vi "CompensateTRY.vi"(0 "Right Wheel Setpoint":dbl, 1 "LeftDriveRefNum":string="My Encoder RefNum", 2 "Try":bool, 3 "Left Wheel Setpoint":dbl, 4 "RightDriveRefNum":string="My Encoder RefNum") -> (5 "Right Wheel Setpoint Out":dbl, 7 "Left Wheel Setpoint Out":dbl)   [LabVIEW 2014]
uses:
  <vilib>/addons/control/pid/pid.llb/PID (DBL).vi
  <vilib>/addons/control/pid/NI_PID_pid.lvlib
panel:
  out "compensate 2":dbl(graph)
  out "compensate 1":dbl(graph)
  out "Dist 2":dbl(graph)
  out "Dist 1":dbl(graph)
  in  "PID gains for motor gain":T1={"proportional gain (Kc)"=1.0, "integral time (Ti, min)"=0.01, "derivative time (Td, min)"=0.0} {"derivative time (Td, min)" format="%.3f"; "integral time (Ti, min)" format="%.3f"; "proportional gain (Kc)" format="%.3f"}
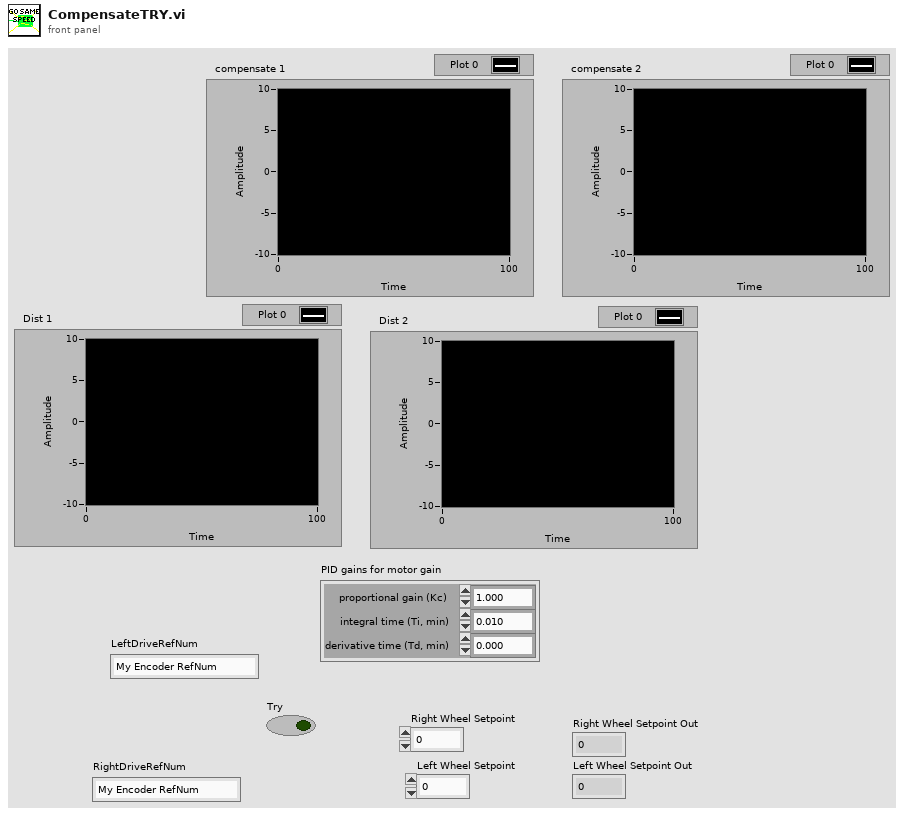
[diagram p1: front panel]
types:
  T1 = cluster{"proportional gain (Kc)":dbl, "integral time (Ti, min)":dbl, "derivative time (Td, min)":dbl}
  T2 = typedef "WPI_EncoderDevRef.ctl" = cluster{"DevStatus":errorcluster, "EncoderIndex":T3, "CounterIndex":T4, "DistancePerCount":dbl, "Decoding Type":T5}
  T3 = typedef "FPGA_EncoderIdx.ctl" = enum8{"Enc 0", "Enc 1", "Enc 2", "Enc 3", "Enc 4", "Enc 5", "Enc 6", "Enc 7", "Invalid"}
  T4 = typedef "FPGA_CounterCtrSystemIndex.ctl" = enum8{"Ctr 0", "Ctr 1", "Ctr 2", "Ctr 3", "Ctr 4", "Ctr 5", "Ctr 6", "Ctr 7", "Invalid"}
  T5 = typedef "WPI_EncoderType.ctl" = enum16{"1x", "2x", "4x"}
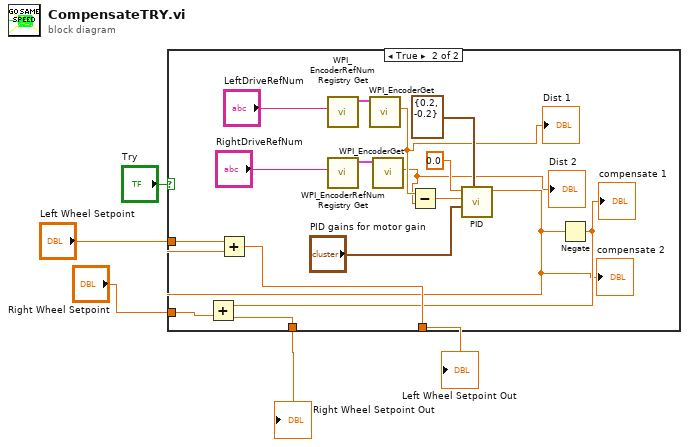
[diagram p0: block diagram]
diagram:
  n1 = case shown="True" "Try" {
    tunnel: "Right Wheel Setpoint" -> [w6 w15]
    tunnel: [w6 w14] -> w3
    tunnel: "Left Wheel Setpoint" -> [w7 w13]
    tunnel: [w7 w12] -> w2
    frame False {
    }
    frame True {
      n2 = call <vilib>:"WPI_EncoderRefNum Registry Get.vi"("refnum name"="LeftDriveRefNum") -> ("EncoderDevRef"=w22:T2)  [unwired: 9 in, 1 out]
      n3 = call <vilib>:"WPI_EncoderRefNum Registry Get.vi"("refnum name"="RightDriveRefNum") -> ("EncoderDevRef"=w19:T2)  [unwired: 9 in, 1 out]
      n4 = call <vilib>:"WPI_EncoderGet.vi"("EncoderDevRef"=w22) -> ("Distance"=w9:dbl)  [unwired: 5 in, 5 out]
      "Dist 1" <- w9
      n5 = call <vilib>:"WPI_EncoderGet.vi"("EncoderDevRef"=w19) -> ("Distance"=w8:dbl)  [unwired: 5 in, 5 out]
      "Dist 2" <- w8
      n6 = Subtract(x=w9, y=w8) -> (x-y=w16:dbl)
      n7 = call-poly <vilib>:"PID.vi"("output range"=cluster{"output high":dbl, "output low":dbl} {"output high"=0.2, "output low"=-0.2}, "PID gains"="PID gains for motor gain", "process variable"=w16, "setpoint"=0.0) -> ("output"=w10:dbl)  [unwired: 6 in, 1 out]
      "compensate 2" <- w10
      n8 = Add(x=w13, y=w10) -> (x+y=w12:dbl)
      n9 = Negate(x=w10) -> (-x=w11:dbl)
      "compensate 1" <- w11
      n10 = Add(x=w11, y=w15) -> (x+y=w14:dbl)
    }
  }
  "Right Wheel Setpoint Out" <- w3
  "Left Wheel Setpoint Out" <- w2
